vi "HandleAbortSync.vi"(8 "error in (no error)":errorcluster, 11 "S4GUI in":refnum<class "S4GUI.lvclass">) -> (0 "error out":errorcluster, 3 "S4GUI out":refnum<class "S4GUI.lvclass">)   [LabVIEW 2018, in "S4GUI.lvclass"]
uses:
  S4GUI.lvclass
  S4GUI.lvclass/S4GUI.ctl
  Instrument/Instrument.lvclass/Instrument.ctl
  Acquisition/Acquisition.lvclass
  Instrument/Instrument.lvclass
  Device/Optics/Opt_Selector/Opt_Selector.lvclass
  Channel/Channel.lvclass
  StateMachine/State Machine.lvclass
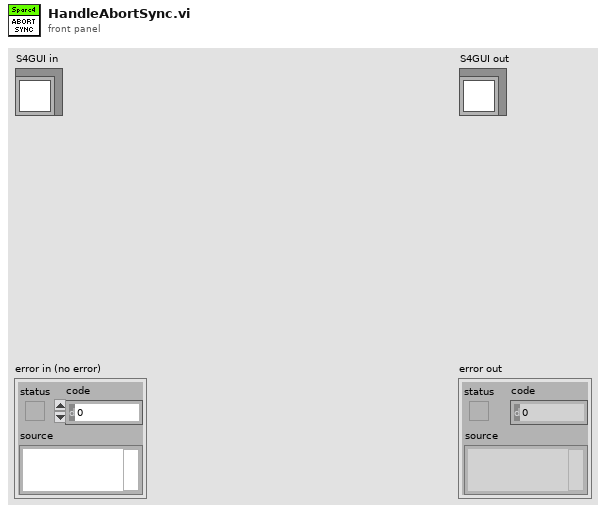
[diagram p1: front panel]
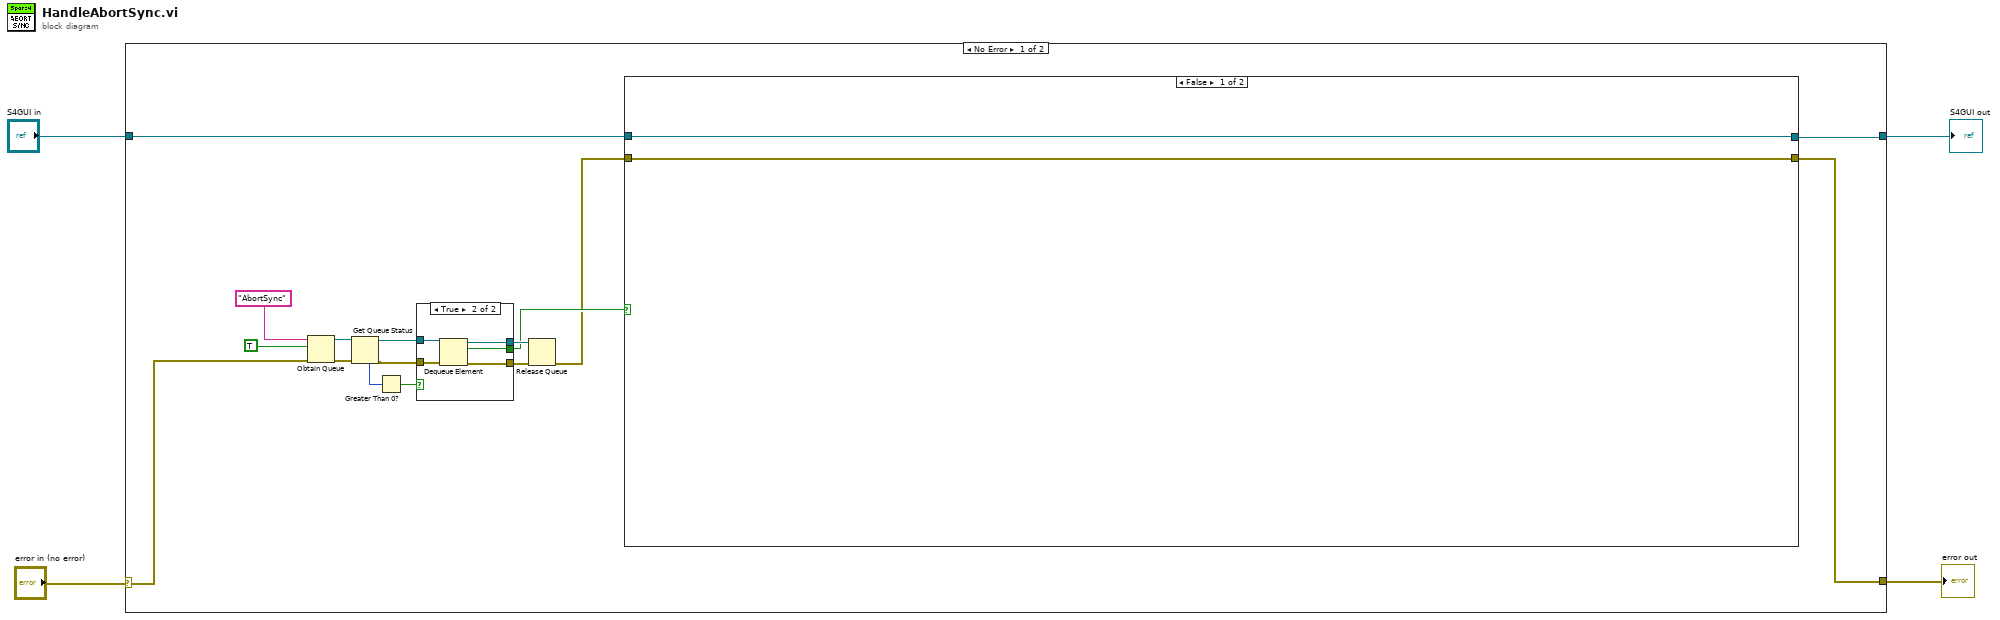
[diagram p0: block diagram]
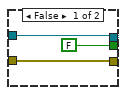
[diagram p2: hidden frame]
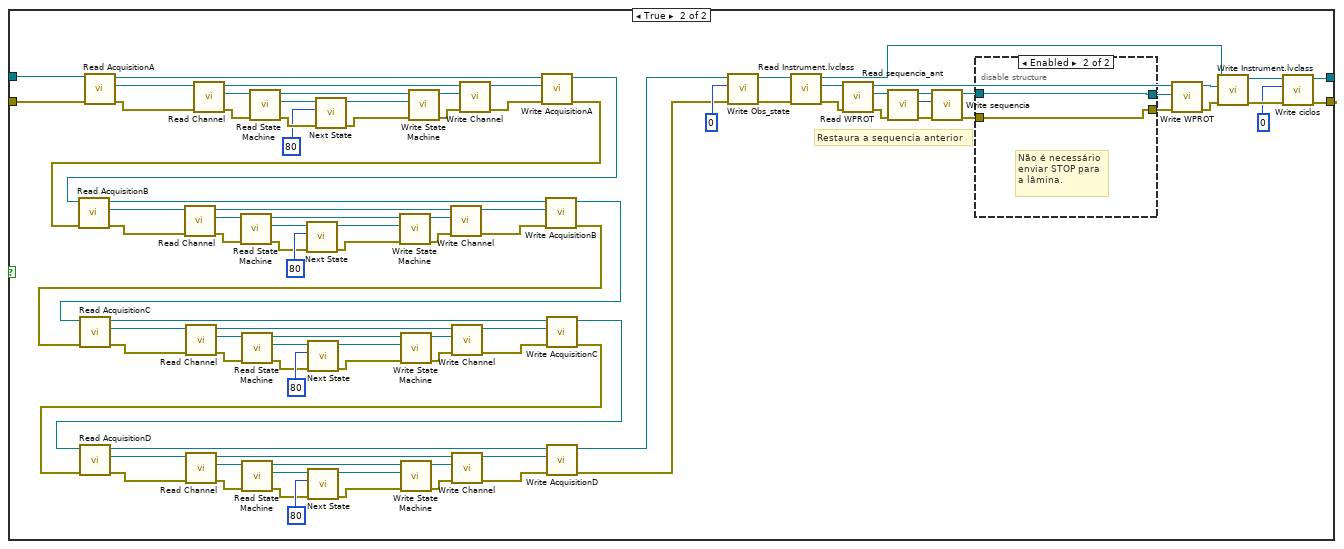
[diagram p3: hidden frame]
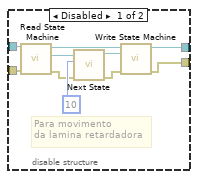
[diagram p4: hidden frame]
diagram:
  n1 = case shown="No Error" "error in (no error)" {
    selector: "error in (no error)" -> [w7 w141]
    tunnel: [w6 w141] -> w3
    tunnel: [w5 w140] -> w1
    tunnel: "S4GUI in" -> [w8 w140]
    frame No Error {
      n2 = Obtain Queue(name (unnamed)="AbortSync", element data type=TRUE, error in (no error)=w7) -> (queue out=w17:refnum<queue>, error out=w18:errorcluster)  [unwired: 2 in, 1 out]
      n3 = Get Queue Status(queue=w17, error in (no error)=w18) -> (queue out=w14:refnum<queue>, error out=w13:errorcluster, # elements in queue=w16:i32)  [unwired: 1 in, 5 out]
      n4 = Greater Than 0?(x=w16) -> (x > 0?=w15:bool)
      n5 = case shown="True" w15 {
        tunnel: w14 -> [w22 w27]
        tunnel: w13 -> [w21 w28]
        tunnel: [FALSE w26] -> w10
        tunnel: [w22 w25] -> w12
        tunnel: [w21 w24] -> w11
        frame False {
        }
        frame True {
          n6 = Dequeue Element(queue=w27, error in (no error)=w28) -> (queue out=w25:refnum<queue>, element=w26:bool, error out=w24:errorcluster)  [unwired: 1 in, 1 out]
        }
      }
      n7 = Release Queue(queue=w12, error in (no error)=w11) -> (error out=w9:errorcluster)  [unwired: 1 in, 2 out]
      n8 = case shown="False" w10 {
        tunnel: w9 -> [w29 w54]
        tunnel: w8 -> [w30 w53]
        tunnel: [w29 w31] -> w6
        tunnel: [w30 w32] -> w5
        frame False {
        }
        frame True {
          # "Restaura a sequencia anterior"
          n9 = call-dynamic "Read AcquisitionA.vi"("error in (no error)"=w54, "S4ACS_GUI in"=w53) -> ("error out"=w115:errorcluster, "Acquisition.lvclass"=w114:refnum<class "Acquisition.lvclass">, "S4ACS_GUI out"=w112:refnum<class "S4GUI.lvclass">)  [unwired: 7 in]
          n10 = call-dynamic "Read Channel.vi"("error in (no error)"=w115, "Acquisition in"=w114) -> ("error out"=w117:errorcluster, "Channel.lvclass"=w116:refnum<class "Channel.lvclass">, "Acquisition out"=w125:refnum<class "Acquisition.lvclass">)  [unwired: 7 in]
          n11 = call-dynamic "Read State Machine.vi"("error in (no error)"=w117, "Device in"=w116) -> ("error out"=w119:errorcluster, "State Machine.lvclass"=w118:refnum<class "State Machine.lvclass">, "Device out"=w121:refnum<class "Channel.lvclass">)  [unwired: 7 in]
          n12 = call "Next State.vi"("error in (no error)"=w119, "New_State"=u32 80, "State Machine in"=w118) -> ("error out"=w122:errorcluster, "State Machine out"=w120:refnum<class "State Machine.lvclass">)  [unwired: 7 in]
          n13 = call-dynamic "Write State Machine.vi"("error in (no error)"=w122, "State Machine.lvclass"=w120, "Device in"=w121) -> ("error out"=w126:errorcluster, "Device out"=w127:refnum<class "Channel.lvclass">)  [unwired: 7 in]
          n14 = call-dynamic "Write Channel.vi"("error in (no error)"=w126, "Channel.lvclass"=w127, "Acquisition in"=w125) -> ("error out"=w124:errorcluster, "Acquisition out"=w123:refnum<class "Acquisition.lvclass">)  [unwired: 7 in]
          n15 = call-dynamic "Write AcquisitionA.vi"("error in (no error)"=w124, "Acquisition.lvclass"=w123, "S4ACS_GUI in"=w112) -> ("error out"=w100:errorcluster, "S4ACS_GUI out"=w99:refnum<class "S4GUI.lvclass">)  [unwired: 7 in]
          n16 = call "Read AcquisitionB.vi"("error in (no error)"=w100, "S4ACS_GUI in"=w99) -> ("error out"=w93:errorcluster, "Acquisition.lvclass"=w97:refnum<class "Acquisition.lvclass">, "S4ACS_GUI out"=w98:refnum<class "S4GUI.lvclass">)  [unwired: 7 in]
          n17 = call-dynamic "Read Channel.vi"("error in (no error)"=w93, "Acquisition in"=w97) -> ("error out"=w108:errorcluster, "Channel.lvclass"=w109:refnum<class "Channel.lvclass">, "Acquisition out"=w95:refnum<class "Acquisition.lvclass">)  [unwired: 7 in]
          n18 = call-dynamic "Read State Machine.vi"("error in (no error)"=w108, "Device in"=w109) -> ("error out"=w106:errorcluster, "State Machine.lvclass"=w107:refnum<class "State Machine.lvclass">, "Device out"=w104:refnum<class "Channel.lvclass">)  [unwired: 7 in]
          n19 = call "Next State.vi"("error in (no error)"=w106, "New_State"=u32 80, "State Machine in"=w107) -> ("error out"=w103:errorcluster, "State Machine out"=w105:refnum<class "State Machine.lvclass">)  [unwired: 7 in]
          n20 = call-dynamic "Write State Machine.vi"("error in (no error)"=w103, "State Machine.lvclass"=w105, "Device in"=w104) -> ("error out"=w102:errorcluster, "Device out"=w101:refnum<class "Channel.lvclass">)  [unwired: 7 in]
          n21 = call-dynamic "Write Channel.vi"("error in (no error)"=w102, "Channel.lvclass"=w101, "Acquisition in"=w95) -> ("error out"=w94:errorcluster, "Acquisition out"=w96:refnum<class "Acquisition.lvclass">)  [unwired: 7 in]
          n22 = call "Write AcquisitionB.vi"("error in (no error)"=w94, "Acquisition.lvclass"=w96, "S4ACS_GUI in"=w98) -> ("error out"=w60:errorcluster, "S4ACS_GUI out"=w59:refnum<class "S4GUI.lvclass">)  [unwired: 7 in]
          n23 = call-dynamic "Read AcquisitionC.vi"("error in (no error)"=w60, "S4ACS_GUI in"=w59) -> ("error out"=w77:errorcluster, "Acquisition.lvclass"=w81:refnum<class "Acquisition.lvclass">, "S4ACS_GUI out"=w82:refnum<class "S4GUI.lvclass">)  [unwired: 7 in]
          n24 = call-dynamic "Read Channel.vi"("error in (no error)"=w77, "Acquisition in"=w81) -> ("error out"=w90:errorcluster, "Channel.lvclass"=w91:refnum<class "Channel.lvclass">, "Acquisition out"=w79:refnum<class "Acquisition.lvclass">)  [unwired: 7 in]
          n25 = call-dynamic "Read State Machine.vi"("error in (no error)"=w90, "Device in"=w91) -> ("error out"=w88:errorcluster, "State Machine.lvclass"=w89:refnum<class "State Machine.lvclass">, "Device out"=w86:refnum<class "Channel.lvclass">)  [unwired: 7 in]
          n26 = call "Next State.vi"("error in (no error)"=w88, "New_State"=u32 80, "State Machine in"=w89) -> ("error out"=w85:errorcluster, "State Machine out"=w87:refnum<class "State Machine.lvclass">)  [unwired: 7 in]
          n27 = call-dynamic "Write State Machine.vi"("error in (no error)"=w85, "State Machine.lvclass"=w87, "Device in"=w86) -> ("error out"=w84:errorcluster, "Device out"=w83:refnum<class "Channel.lvclass">)  [unwired: 7 in]
          n28 = call-dynamic "Write Channel.vi"("error in (no error)"=w84, "Channel.lvclass"=w83, "Acquisition in"=w79) -> ("error out"=w78:errorcluster, "Acquisition out"=w80:refnum<class "Acquisition.lvclass">)  [unwired: 7 in]
          n29 = call-dynamic "Write AcquisitionC.vi"("error in (no error)"=w78, "Acquisition.lvclass"=w80, "S4ACS_GUI in"=w82) -> ("error out"=w58:errorcluster, "S4ACS_GUI out"=w57:refnum<class "S4GUI.lvclass">)  [unwired: 7 in]
          n30 = call-dynamic "Read AcquisitionD.vi"("error in (no error)"=w58, "S4ACS_GUI in"=w57) -> ("error out"=w61:errorcluster, "Acquisition.lvclass"=w65:refnum<class "Acquisition.lvclass">, "S4ACS_GUI out"=w66:refnum<class "S4GUI.lvclass">)  [unwired: 7 in]
          n31 = call-dynamic "Read Channel.vi"("error in (no error)"=w61, "Acquisition in"=w65) -> ("error out"=w74:errorcluster, "Channel.lvclass"=w75:refnum<class "Channel.lvclass">, "Acquisition out"=w63:refnum<class "Acquisition.lvclass">)  [unwired: 7 in]
          n32 = call-dynamic "Read State Machine.vi"("error in (no error)"=w74, "Device in"=w75) -> ("error out"=w72:errorcluster, "State Machine.lvclass"=w73:refnum<class "State Machine.lvclass">, "Device out"=w70:refnum<class "Channel.lvclass">)  [unwired: 7 in]
          n33 = call "Next State.vi"("error in (no error)"=w72, "New_State"=u32 80, "State Machine in"=w73) -> ("error out"=w69:errorcluster, "State Machine out"=w71:refnum<class "State Machine.lvclass">)  [unwired: 7 in]
          n34 = call-dynamic "Write State Machine.vi"("error in (no error)"=w69, "State Machine.lvclass"=w71, "Device in"=w70) -> ("error out"=w68:errorcluster, "Device out"=w67:refnum<class "Channel.lvclass">)  [unwired: 7 in]
          n35 = call-dynamic "Write Channel.vi"("error in (no error)"=w68, "Channel.lvclass"=w67, "Acquisition in"=w63) -> ("error out"=w62:errorcluster, "Acquisition out"=w64:refnum<class "Acquisition.lvclass">)  [unwired: 7 in]
          n36 = call-dynamic "Write AcquisitionD.vi"("error in (no error)"=w62, "Acquisition.lvclass"=w64, "S4ACS_GUI in"=w66) -> ("error out"=w55:errorcluster, "S4ACS_GUI out"=w56:refnum<class "S4GUI.lvclass">)  [unwired: 7 in]
          n37 = call-dynamic "Write Obs_state.vi"("error in (no error)"=w55, "Obs_state"=u32 0, "S4ACS_GUI in"=w56) -> ("error out"=w33:errorcluster, "S4ACS_GUI out"=w34:refnum<class "S4GUI.lvclass">)  [unwired: 7 in]
          n38 = call "Read Instrument.lvclass.vi"("error in (no error)"=w33, "S4ACS_GUI in"=w34) -> ("error out"=w47:errorcluster, "Instrument.lvclass"=w49:refnum<class "Instrument.lvclass">, "S4ACS_GUI out"=w48:refnum<class "S4GUI.lvclass">)  [unwired: 7 in]
          n39 = call "Read WPROT.vi"("error in (no error)"=w47, "Instrument in"=w49) -> ("error out"=w42:errorcluster, "Opt_Selector.lvclass"=w45:refnum<class "Opt_Selector.lvclass">, "Instrument out"=w50:refnum<class "Instrument.lvclass">)  [unwired: 7 in]
          n40 = call-dynamic "Read sequencia_ant.vi"("error in (no error)"=w42, "Opt_Selector in"=w45) -> ("error out"=w41:errorcluster, "sequencia_ant"=w43:u16, "Opt_Selector out"=w44:refnum<class "Opt_Selector.lvclass">)  [unwired: 7 in]
          n41 = call-dynamic "Write sequencia.vi"("error in (no error)"=w41, "sequencia"=w43, "Opt_Selector in"=w44) -> ("error out"=w39:errorcluster, "Opt_Selector out"=w40:refnum<class "Opt_Selector.lvclass">)  [unwired: 7 in]
          n42 = disable-structure shown="Enabled" {
            disable-tunnel: w40 -> [w134 w139]
            disable-tunnel: w39 -> [w133 w138]
            disable-tunnel: [w129 w138] -> w38
            disable-tunnel: [w128 w139] -> w37
            frame Disabled {
              # "Para movimento \nda lamina retardadora"
              n43 = call-dynamic "Read State Machine.vi"("error in (no error)"=w133, "Device in"=w134) -> ("error out"=w136:errorcluster, "State Machine.lvclass"=w131:refnum<class "State Machine.lvclass">, "Device out"=w132:refnum<class "Opt_Selector.lvclass">)  [unwired: 7 in]
              n44 = call "Next State.vi"("error in (no error)"=w136, "New_State"=10, "State Machine in"=w131) -> ("error out"=w135:errorcluster, "State Machine out"=w130:refnum<class "State Machine.lvclass">)  [unwired: 7 in]
              n45 = call-dynamic "Write State Machine.vi"("error in (no error)"=w135, "State Machine.lvclass"=w130, "Device in"=w132) -> ("error out"=w129:errorcluster, "Device out"=w128:refnum<class "Opt_Selector.lvclass">)  [unwired: 7 in]
            }
            frame Enabled {
              # "Não é necessário\nenviar STOP para\na lâmina."
            }
          }
          n46 = call "Write WPROT.vi"("error in (no error)"=w38, "Opt_Selector.lvclass"=w37, "Instrument in"=w50) -> ("error out"=w35:errorcluster, "Instrument out"=w36:refnum<class "Instrument.lvclass">)  [unwired: 7 in]
          n47 = call "Write Instrument.lvclass.vi"("error in (no error)"=w35, "Instrument.lvclass"=w36, "S4ACS_GUI in"=w48) -> ("error out"=w51:errorcluster, "S4ACS_GUI out"=w52:refnum<class "S4GUI.lvclass">)  [unwired: 7 in]
          n48 = call-dynamic "Write ciclos.vi"("error in (no error)"=w51, "ciclos"=u32 0, "S4ACS_GUI in"=w52) -> ("error out"=w31:errorcluster, "S4ACS_GUI out"=w32:refnum<class "S4GUI.lvclass">)  [unwired: 7 in]
        }
      }
    }
    frame Error {
    }
  }
  "error out" <- w3
  "S4GUI out" <- w1
